vi "HC-SR04 ile park sensoru.vi"() -> ()   [LabVIEW 2018]
doc: "This example performs writes and reads on a serial port, as directed by the user. You can press the Write and Read buttons, and change the Read Count, while the example is running.\n\nThe parameters set for the serial port must match the parameters of the connected instrument or device. In this example, the Read Count parameter specifies the number of bytes that the serial port reads. If there were more bytes at the port than the specified number, those bytes would not be read. If there were less bytes at the port than the specified number, you would receive a timeout error.\n\nThis example expands upon the flow control options for XON and XOFF, allowing the user to choose those control characters. Also, the user can enable or disable a termination character. Some devices require a termination character in order to identify the end of command strings. Some devices send a termination character to signify the end of data to be read. This example shows how you can end the Read operation once a termination character is detected in the buffer and/or append a termination character at the end of the Write data."
uses:
  Program Files (x86)/National Instruments/LabVIEW 2018/examples/Instrument IO/Serial/support/Serial - Settings.ctl
  Program Files (x86)/National Instruments/LabVIEW 2018/examples/Instrument IO/Serial/support/Serial - XON-XOFF Characters.ctl
  Program Files (x86)/National Instruments/LabVIEW 2018/examples/Instrument IO/Serial/support/Serial - ASCII Characters.ctl
  <vilib>/Instr/_visa.llb/VISA Configure Serial Port (Instr).vi
panel:
  out "Gauge 2":dbl(knob) scale=0.0..400.0
  in  "Termination Character":u8=10 format="%.0x"
  in  "Stop":bool
  in  "Read Count":u32=1000
  out "Response":string
  in  "XON/XOFF Characters":T1={"XON"=enum."DC1", "XOFF"=enum."DC3"}
  in  "Serial Settings":T3={"baud rate"=9600, "data bits"=8, "parity"=enum."None", "stop bits"=10, "flow control"=0} {"flow control" items=["None"=0, "XON/XOFF"=1, "RTS/CTS"=2, "DTR/DSR"=4]; "stop bits" items=["1.0"=10, "1.5"=15, "2.0"=20]; "data bits" min=5 max=8 step=1; "baud rate" items=["75"=75, "110"=110, "134"=134, "150"=150, "300"=300, "600"=600, "1200"=1200, "1800"=1800, "2400"=2400, "4800"=4800, "7200"=7200, "9600"=9600, "14400"=14400, "19200"=19200, "28800"=28800, "38400"=38400, "56000"=56000, "57600"=57600, "115200"=115200, "128000"=128000, "230400"=230400]}
  in  "End Read on Termination Character?":bool=TRUE
  in  "VISA resource name":refnum<visa-resource-name>="COM1"
  # "HC-SR04 İLE PARK SENSÖRÜ"
  # "AYARLAR"
  # "GÖSTERGE PANELİ"
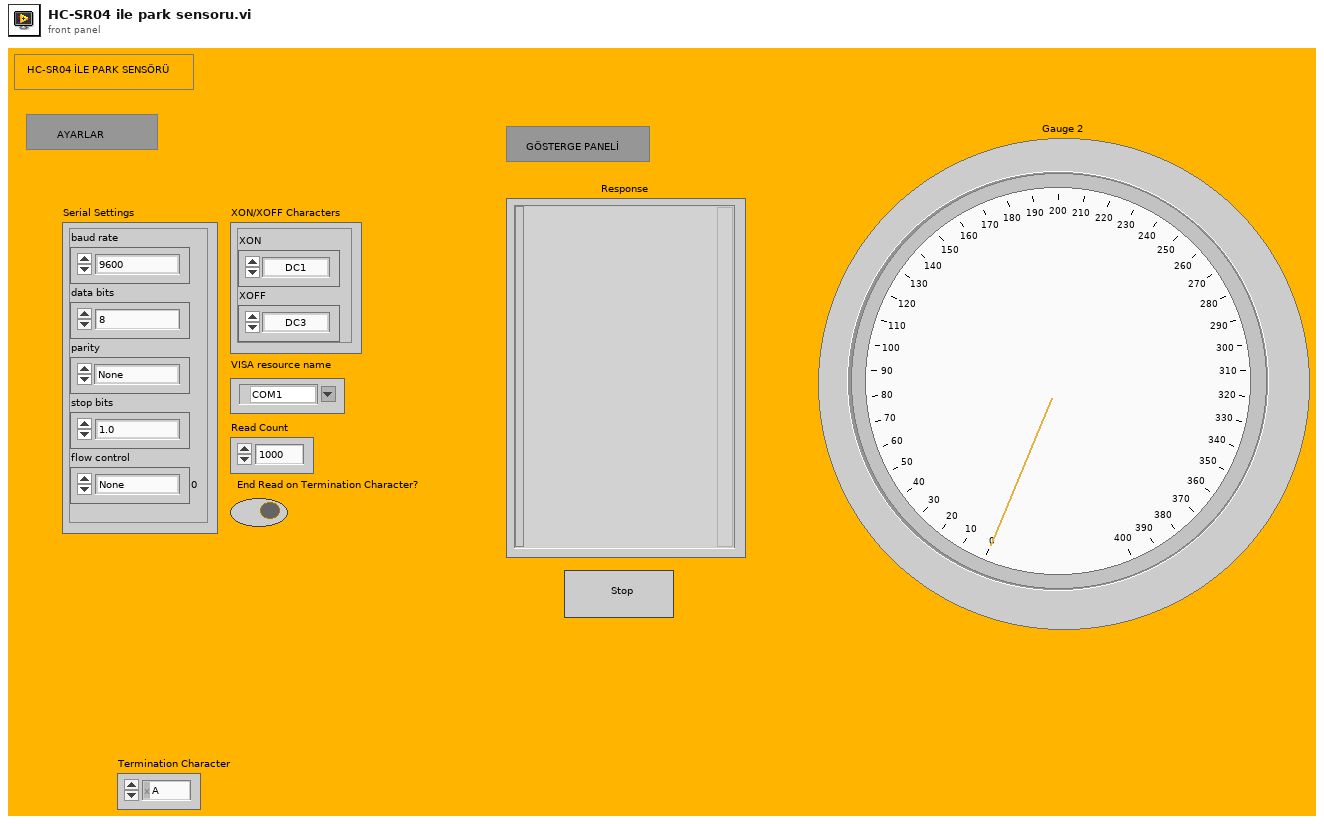
[diagram p1: front panel]
types:
  T1 = typedef "Serial - XON-XOFF Characters.ctl" = cluster{"XON":T2, "XOFF":T2}
  T2 = typedef "Serial - ASCII Characters.ctl" = enum16{"NUL", "SOH", "STX", "ETX", "EOT", "ENQ", "ACK", "BEL", "BS", "HT", "LF", "VT", "FF", "CR", "SO", "SI", "DLE", "DC1", "DC2", "DC3", "DC4", "NAK", "SYN", "ETB", "CAN", "EM", "SUB", "ESC", "FS", "GS", "RS", "US", "SP", "!", "\"", "#", "$", "%", "&", "'", "(", ")", "*", "+", ",", "- (-)", ".", "/", "0", "1", "2", "3", "4", "5", "6", "7", "8", "9", ":", ";", "<", "=", ">", "?", "@", "A", "B", "C", "D", "E", "F", "G", "H", "I", "J", "K", "L", "M", "N", "O", "P", "Q", "R", "S", "T", "U", "V", "W", "X", "Y", "Z", "[", "\\", "]", "^", "_", "`", "a", "b", "c", "d", "e", "f", "g", "h", "i", "j", "k", "l", "m", "n", "o", "p", "q", "r", "s", "t", "u", "v", "w", "x", "y", "z", "{", "|", "}", "~"}
  T3 = typedef "Serial - Settings.ctl" = cluster{"baud rate":u32, "data bits":u16, "parity":enum16{"None", "Odd", "Even", "Mark", "Space"}, "stop bits":u16, "flow control":u16}
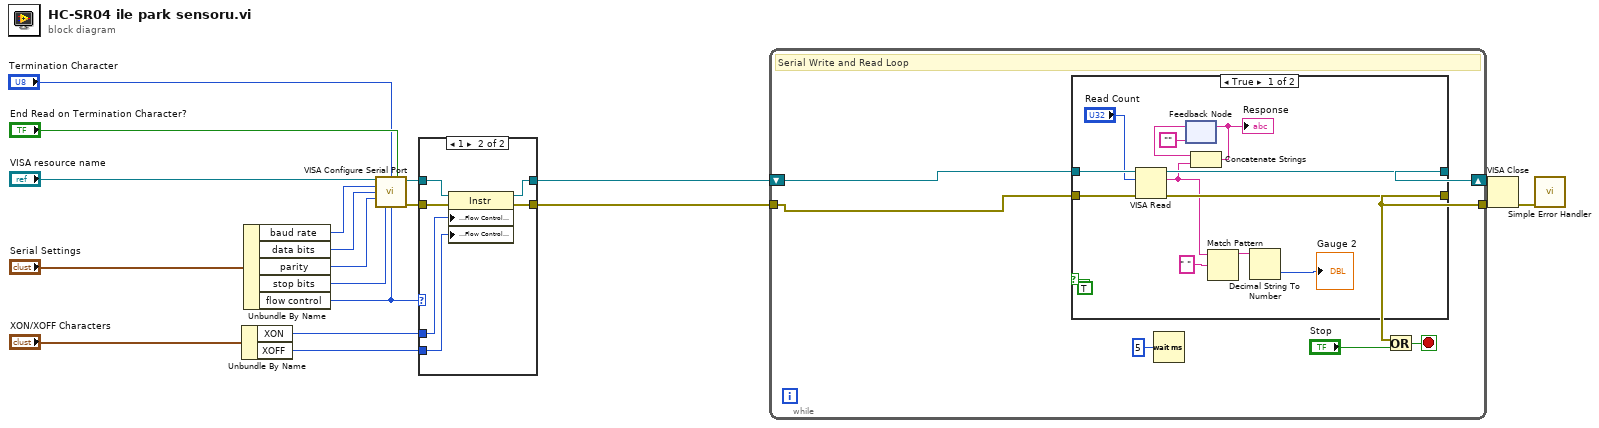
[diagram p0: block diagram]
diagram:
  n1 = Unbundle By Name("XON/XOFF Characters") -> ("XON"=w5:T2, "XOFF"=w4:T2)
  n2 = Unbundle By Name("Serial Settings") -> ("baud rate"=w12:u32, "data bits"=w13:u16, "parity"=w14:enum16{"None", "Odd", "Even", "Mark", "Space"}, "stop bits"=w15:u16, "flow control"=w6:u16)
  n3 = call-poly "VISA Configure Serial Port"("VISA resource name"="VISA resource name", "termination char\n(0xA = '\\n' = LF)"="Termination Character", "Enable Termination\nChar (T)"="End Read on Termination Character?", "baud rate (9600)"=w12, "data bits (8)"=w13, "parity (0:none)"=w14, "stop bits (10: 1 bit)"=w15, "flow control (0:none)"=w6) -> ("VISA resource name out"=w16:refnum<visa-resource-name>, "error out"=w17:errorcluster)  [unwired: 2 in, 4 out]
  n4 = case shown="1" w6 {
    tunnel: [w20 w27] -> w1
    tunnel: [w21 w26] -> w2
    tunnel: w17 -> [w20 w25]
    tunnel: w16 -> [w21 w24]
    tunnel: w5 -> [_ w23]
    tunnel: w4 -> [_ w22]
    frame Default {
    }
    frame 1 {
      n5 = property class="Instr"(reference=w24, error in=w25, "Serial Settings:Flow Control XON Character"=w23, "Serial Settings:Flow Control XOFF Character"=w22) -> (reference out=w26:refnum<visa-resource-name>, error out=w27:errorcluster)
    }
  }
  n6 = while {
    shift-right: [w35] -> w7
    shift-left: w2 -> [w30]
    tunnel: w1 -> [w29]
    tunnel: [w32] -> w8
    stop <- w33 stop-if-true
    # "Serial Write and Read Loop"
    n7 = case shown="True" TRUE {
      tunnel: [w45 w49] -> w35
      tunnel: w30 -> [w47 w49]
      tunnel: [w43 w48] -> w32
      tunnel: w29 -> [w46 w48]
      frame True {
        n8 = VISA Read(VISA resource name=w47, byte count="Read Count", error in (no error)=w46) -> (VISA resource name out=w45:refnum<visa-resource-name>, read buffer=w37:string, error out=w43:errorcluster)  [unwired: 1 out]
        n9 = feedback #1("") -> (w42:string)
        n10 = Concatenate Strings(w42, w37) -> (w41:string)
        "Response" <- w41
        n11 = feedback-in #1(w41) -> ()
        n12 = Match Pattern(string=w37, regular expression=" ") -> (before substring=w38:string)  [unwired: 1 in, 3 out]
        n13 = Decimal String To Number(string=w38) -> (number=→"Gauge 2":i32)  [unwired: 2 in, 1 out]
      }
      frame False {
      }
    }
    n14 = Wait (ms)(milliseconds to wait=u32 5) -> ()  [unwired: 1 out]
    n15 = Or(x=w32, y="Stop") -> (x .or. y?=w33:bool)
  }
  n16 = VISA Close(VISA resource name=w7, error in (no error)=w8) -> (error out=w9:errorcluster)
  n17 = call <vilib>:"Simple Error Handler.vi"("error in (no error)"=w9) -> ()  [unwired: 1 in, 8 out]
